vi "SRV_PM_Receive State Machine.vi"(7 "Cancelled?":bool, 8 "error in (no error)":errorcluster, 9 "SRV_Packets queue":refnum<queue>, 10 "TCP Read semaphore":T1, 11 "SRV IP Address":string) -> (0 "error out":errorcluster)   [LabVIEW 2009]
doc: "Author: Mike Schultz (LogicPD, Inc)"
uses:
  SRV_PM_Packet.ctl
  Support/SRV_Command-Data Queue Data Type.ctl
  SRV_PM_Receive State Machine Local Data.ctl
  TCP_Communication/SRV_TCP Settings.ctl
  TCP_Communication/SRV_Package Methods.ctl
  <vilib>/Utility/error.llb/DialogType.ctl
panel:
  in  "reset max 3":bool
  out "Evals max":i32
  out "Eval in a row":i32
  out "get ref ms":u32
  out "sema ms":u32
  out "Read 1 ms":u32
  in  "Delay Before Read (ms)":u32
  in  "reset max 2":bool
  out "new size max":i32
  in  "reset max":bool
  out "WIP Size max":i32
  out "Trim ms":u32
  out "New Packet Data size":i32
  out "Build ms":u32
  out "WIP Size":i32
  out "Eval ms":u32
  out "Read ms":u32
  out "Loop ms":u32
  out "ms since last ad":u32
  out "# elements in queue":i32
  out "i":i32
  out "Command History":string[](array[string])
  out "Command":string
  out "Packet Complete?":bool
  out "New Packet Data":u8[](array[numeric]) format="%.0x"
  out "Packet":T2 {"Packet Data" format="%.0x"}
  in  "Use Debug New Packet Data?":bool
  in  "New Packet Data":u8[](array[numeric]) format="%.0x"
  # "Read"
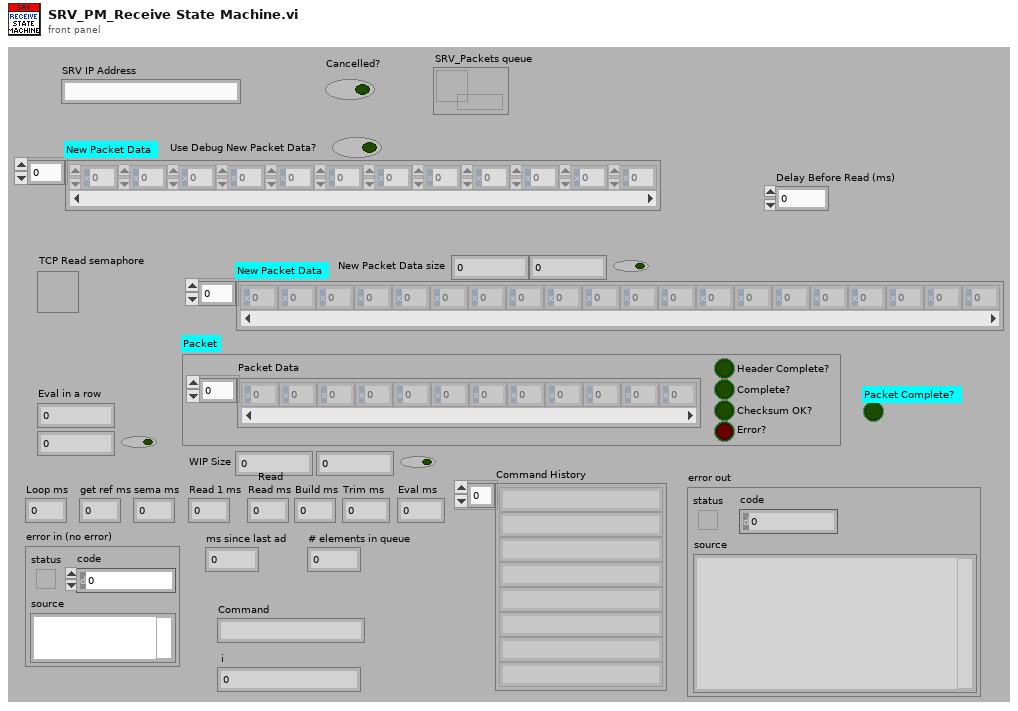
[diagram p1: front panel]
types:
  T1 = typedef "Semaphore RefNum" = refnum<k1>
  T2 = typedef "SRV_PM_Packet.ctl" = cluster{"Packet Data":u8[], "Header Complete?":bool, "Complete?":bool, "Checksum OK?":bool, "Error?":bool}
  T3 = typedef "SRV_PM_Receive State Machine Local Data.ctl" = cluster{"Packet Data WIP":u8[], "New Packet Data":u8[], "Complete Packet":T2, "SRV IP Address":string, "TCP Read semaphore":T1, "SRV_Packets queue":refnum<queue>, "Evals in a row":i32}
  T4 = typedef "SRV_Command-Data Queue Data Type.ctl" = cluster{"Command":string, "Data":variant}
  T5 = typedef "SRV_TCP Settings.ctl" = cluster{"Method":T6, "bytes to read":i32, "timeout ms (1000)":i32}
  T6 = typedef "SRV_Package Methods.ctl" = enum16{"General", "Standard", "CRLF", "Image", "HTML"}
  T7 = typedef "DialogType.ctl" = u16
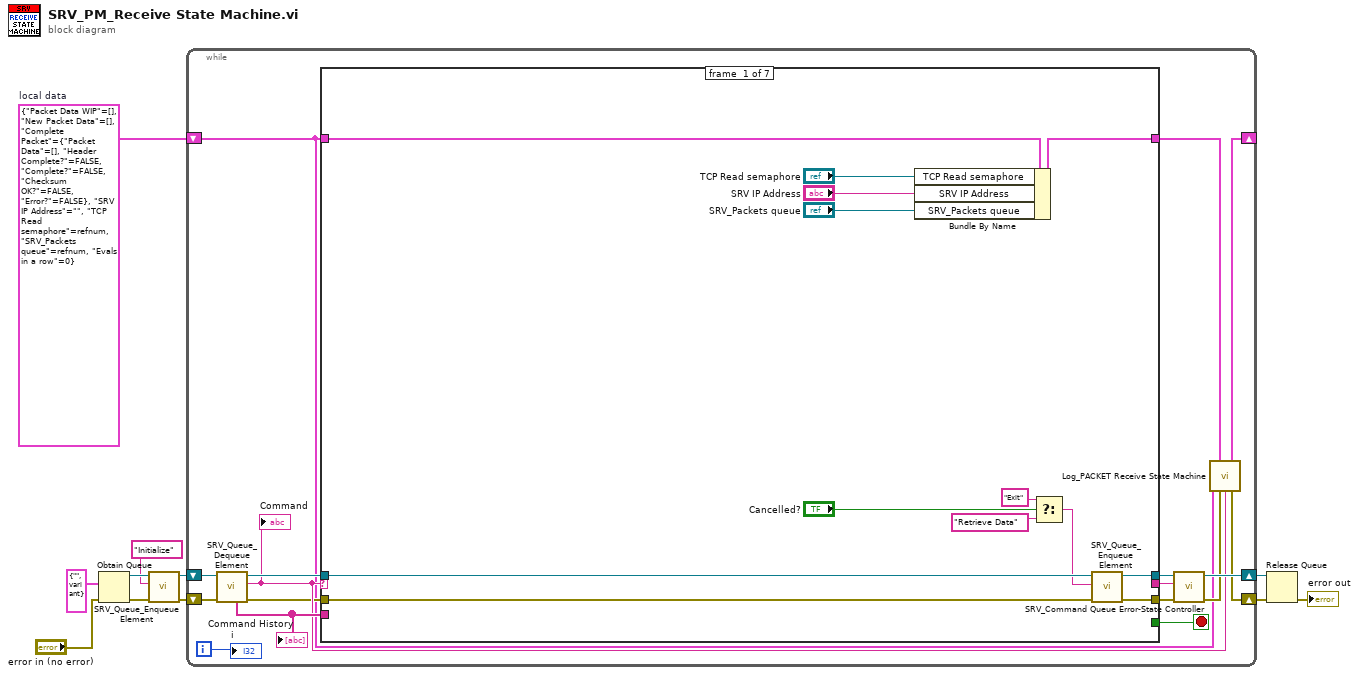
[diagram p0: block diagram]
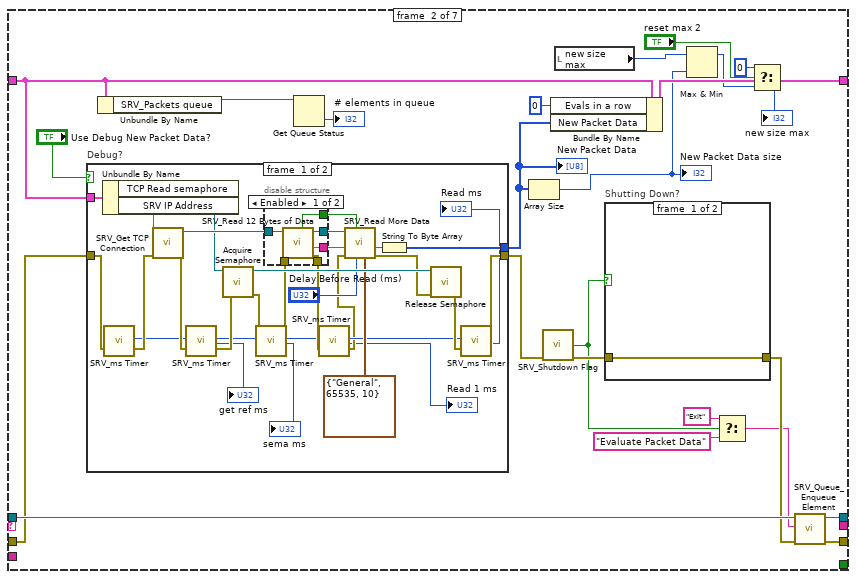
[diagram p2: hidden frame]
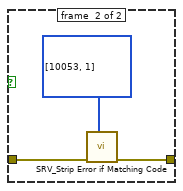
[diagram p3: hidden frame]
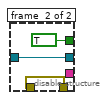
[diagram p4: hidden frame]
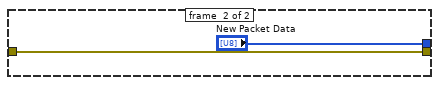
[diagram p5: hidden frame]
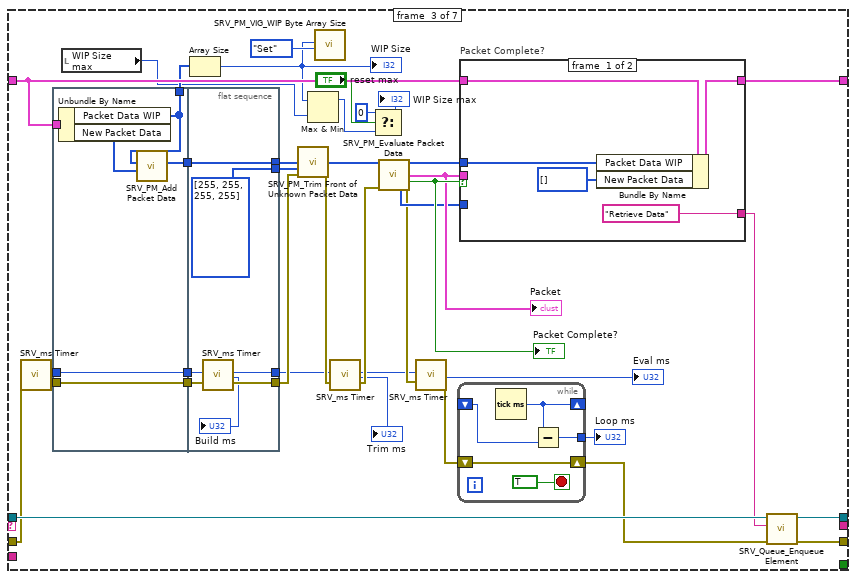
[diagram p6: hidden frame]
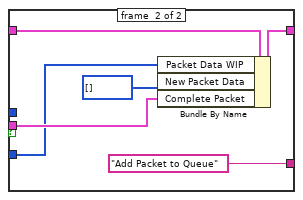
[diagram p7: hidden frame]
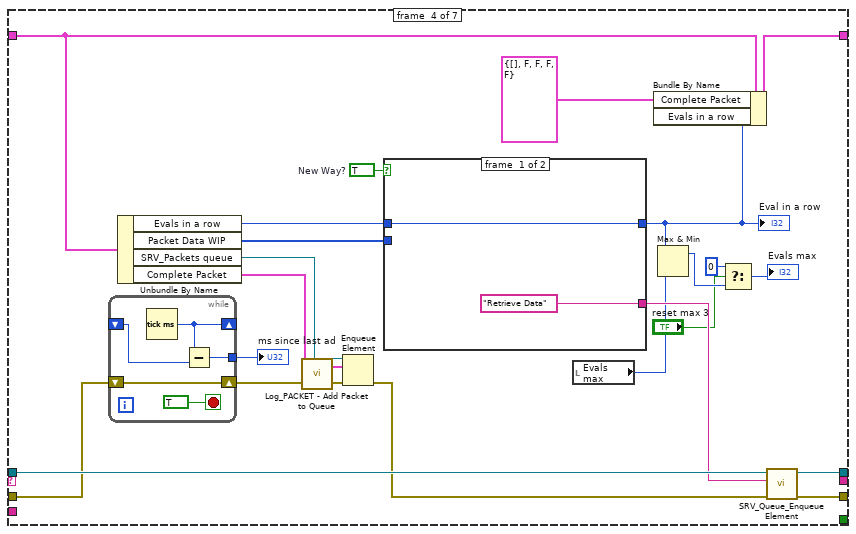
[diagram p8: hidden frame]
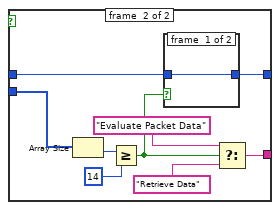
[diagram p9: hidden frame]
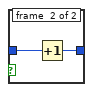
[diagram p10: hidden frame]
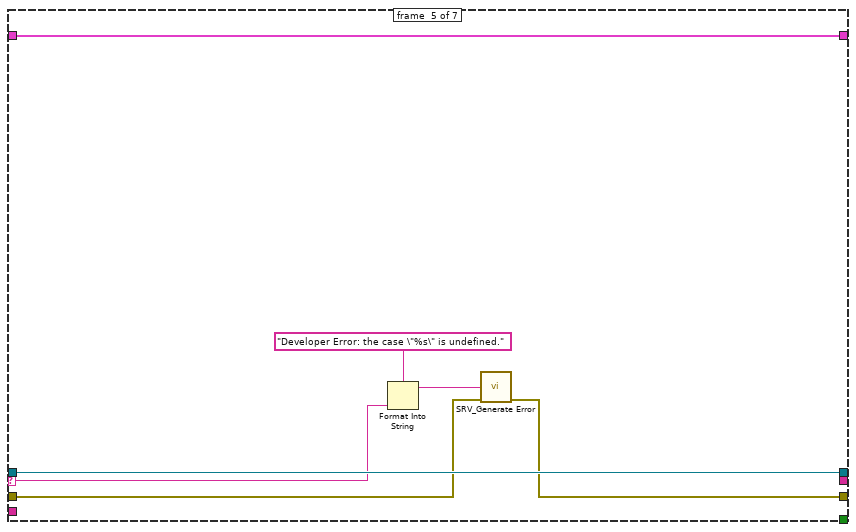
[diagram p11: hidden frame]
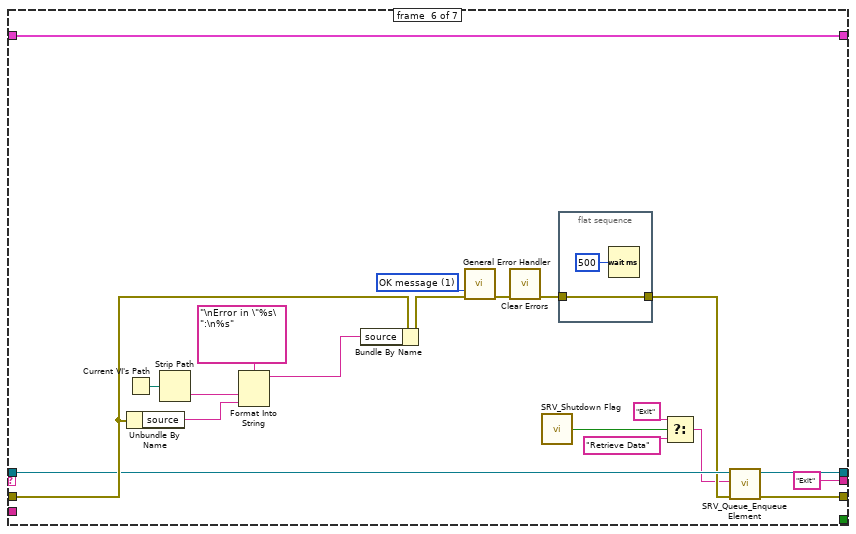
[diagram p12: hidden frame]
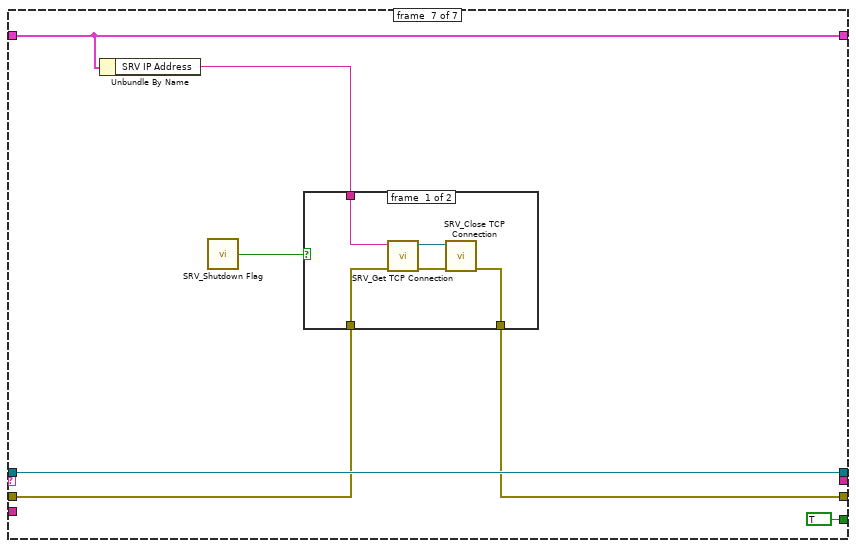
[diagram p13: hidden frame]
diagram:
  w1 = T3 {"Packet Data WIP"=[], "New Packet Data"=[], "Complete Packet"={"Packet Data"=[], "Header Complete?"=FALSE, "Complete?"=FALSE, "Checksum OK?"=FALSE, "Error?"=FALSE}, "SRV IP Address"="", "TCP Read semaphore"=refnum, "SRV_Packets queue"=refnum, "Evals in a row"=0}  # local data
  n1 = Obtain Queue(element data type=T4 {"Command"="", "Data"=variant} ("Queue Data Type"), error in (no error)="error in (no error)") -> (queue out=w10:refnum<queue>, error out=w8:errorcluster)  [unwired: 3 in, 1 out]
  n2 = call "SRV_Queue_Enqueue Element.vi"("error in (no error)"=w8, "Command"="Initialize", "Command-Data Queue"=w10) -> ("error out"=w7:errorcluster, "Command-Data Queue out"=w9:refnum<queue>)  [unwired: 6 in, 1 out]
  n3 = while {
    shift-right: [w17] -> w4
    shift-left: w7 -> [w28]
    shift-right: [w23] -> w5
    shift-left: w9 -> [w27]
    shift-right: [w14] -> _
    shift-left: w1 -> [w12]
    i -> [w19]
    stop <- w25 stop-if-true
    n4 = call "SRV_Queue_Dequeue Element.vi"("error in (no error)"=w28, "Command-Data Queue"=w27) -> ("error out"=w13:errorcluster, "Command"=w16:string, "Command-Data Queue out"=w26:refnum<queue>, "Command History"=w20:string[])  [unwired: 4 in, 2 out]
    "Command" <- w16
    "Command History" <- w20
    n5 = case shown="\"Add Packet to Queue\"" w16 {
      selector: w16 -> [_ _ _ _ w224 _ _]
      tunnel: w13 -> [w35 w61 w128 w194 w226 w238 w254]
      tunnel: [w41 w64 w148 w201 w227 w237 w255] -> w22
      tunnel: [w40 w65 w149 w202 w228 w235 w257] -> w24
      tunnel: w26 -> [w39 w63 w147 w200 w228 w236 w257]
      tunnel: [_ _ _ _ _ _ TRUE] -> w25
      tunnel: [_ _ _ _ _ "Exit" ("Error Command") _] -> w21
      tunnel: w12 -> [w38 w52 w142 w199 w222 w247 w252]
      tunnel: [w37 w62 w146 w198 w222 w247 w252] -> w15
      tunnel: w20 -> [_ _ _ _ _ _ _]
      frame #0 {
        n6 = Bundle By Name(cluster=w38, "TCP Read semaphore"="TCP Read semaphore", "SRV IP Address"="SRV IP Address", "SRV_Packets queue"="SRV_Packets queue") -> (w37:T3)
        n7 = Select(t="Exit" ("Command"), s="Cancelled?", f="Retrieve Data" ("Command")) -> (s? t:f=w31:string)
        n8 = call "SRV_Queue_Enqueue Element.vi"("error in (no error)"=w35, "Command"=w31, "Command-Data Queue"=w39) -> ("error out"=w41:errorcluster, "Command-Data Queue out"=w40:refnum<queue>)  [unwired: 6 in, 1 out]
      }
      frame #1 {
        n9 = case "Debug?" shown="False" "Use Debug New Packet Data?" {
          tunnel: w61 -> [w89 w110]
          tunnel: [w86 w110] -> w59
          tunnel: [w100 "New Packet Data"] -> w49
          tunnel: w52 -> [w94 _]
          frame #0 {
            n10 = Unbundle By Name(w94) -> ("TCP Read semaphore"=w92:T1, "SRV IP Address"=w93:string)
            n11 = call "SRV_ms Timer.vi"("error in (no error)"=w89) -> ("ms Tick"=w74:u32, "error out"=w88:errorcluster)  [unwired: 16 in, 1 out]
            n12 = call "SRV_Get TCP Connection.vi"("error in (no error)"=w88, "IP address"=w93) -> ("error out"=w78:errorcluster, "connection ID"=w95:refnum<k5>)  [unwired: 8 in]
            n13 = call "SRV_ms Timer.vi"("ms Previous Tick"=w74, "error in (no error)"=w78) -> ("ms Tick"=w73:u32, "ms Diff"=→"get ref ms":u32, "error out"=w77:errorcluster)  [unwired: 15 in]
            n14 = call <vilib>:"Acquire Semaphore.vi"("error in (no error)"=w77, "semaphore"=w92) -> ("error out"=w76:errorcluster, "semaphore out"=w91:T1)  [unwired: 3 in, 1 out]
            n15 = call "SRV_ms Timer.vi"("ms Previous Tick"=w73, "error in (no error)"=w76) -> ("ms Tick"=w72:u32, "ms Diff"=→"sema ms":u32, "error out"=w75:errorcluster)  [unwired: 15 in]
            n16 = disable-structure shown="Enabled" {
              disable-tunnel: [w106 TRUE ("Read More Data? (T)")] -> w99
              disable-tunnel: [w105 w108] -> w98
              disable-tunnel: [w104 _] -> w97
              disable-tunnel: w95 -> [w103 w108]
              disable-tunnel: [w102 w109] -> w81
              disable-tunnel: w75 -> [w101 w109]
              frame #0 {
                n17 = call "SRV_Read 12 Bytes of Data.vi"("error in (no error)"=w101, "SRV In"=w103) -> ("error out"=w102:errorcluster, "Data out"=w104:string, "SRV Out"=w105:refnum<k5>, "Read more data"=w106:bool)  [unwired: 6 in]
              }
              frame #1 {
              }
            }
            n18 = call "SRV_ms Timer.vi"("ms Previous Tick"=w72, "error in (no error)"=w81) -> ("ms Tick"=w82:u32, "ms Diff"=→"Read 1 ms":u32, "error out"=w80:errorcluster)  [unwired: 15 in]
            n19 = call "SRV_Read More Data.vi"("TCP Settings"=T5 {"Method"=enum."General", "bytes to read"=65535, "timeout ms (1000)"=10}, "Delay Before Read (10ms)"="Delay Before Read (ms)", "Read More Data? (T)"=w99, "error in (no error)"=w80, "Data in"=w97, "Connection ID"=w98) -> ("error out"=w90:errorcluster, "Data out"=w96:string)  [unwired: 3 in, 1 out]
            n20 = String To Byte Array(string=w96) -> (unsigned byte array=w100:u8[])
            n21 = call <vilib>:"Release Semaphore.vi"("error in (no error)"=w90, "semaphore"=w91) -> ("error out"=w87:errorcluster)  [unwired: 4 in, 1 out]
            n22 = call "SRV_ms Timer.vi"("ms Previous Tick"=w82, "error in (no error)"=w87) -> ("ms Diff"=→"Read ms":u32, "error out"=w86:errorcluster)  [unwired: 15 in, 1 out]
          }
          frame #1 {
          }
        }
        "New Packet Data" <- w49
        n23 = Unbundle By Name(w52) -> ("SRV_Packets queue"=w51:refnum<queue>)
        n24 = Get Queue Status(queue=w51) -> (# elements in queue=→"# elements in queue":i32)  [unwired: 2 in, 7 out]
        n25 = Array Size(array=w49) -> (size(s)=w45:i32)
        "New Packet Data size" <- w45
        n26 = call "SRV_Shutdown Flag.vi"("error in (no error)"=w59) -> ("Shutdown Flag out"=w53:bool, "error out"=w58:errorcluster)  [unwired: 13 in]
        n27 = Bundle By Name(cluster=w52, "Evals in a row"=0, "New Packet Data"=w49) -> (w62:T3)
        n28 = local read "new size max"() -> (w46:i32)
        n29 = case "Shutting Down?" shown="True" w53 {
          tunnel: w58 -> [w66 w69]
          tunnel: [w66 w68] -> w57
          frame #0 {
          }
          frame #1 {
            n30 = call "SRV_Strip Error if Matching Code.vi"("error in (no error)"=w69, "Strip Codes"=i32[] [10053, 1]) -> ("error out"=w68:errorcluster)  [unwired: 8 in]
          }
        }
        n31 = Max & Min(x=w46, y=w45) -> (max(x,y)=w48:i32)  [unwired: 1 out]
        n32 = Select(t="Exit" ("Command"), s=w53, f="Evaluate Packet Data" ("Command")) -> (s? t:f=w55:string)
        n33 = Select(t=0, s="reset max 2", f=w48) -> (s? t:f=→"new size max":i32)
        n34 = call "SRV_Queue_Enqueue Element.vi"("error in (no error)"=w57, "Command"=w55, "Command-Data Queue"=w63) -> ("error out"=w64:errorcluster, "Command-Data Queue out"=w65:refnum<queue>)  [unwired: 6 in, 1 out]
      }
      frame #2 {
        n35 = call "SRV_ms Timer.vi"("error in (no error)"=w128) -> ("ms Tick"=w126:u32, "error out"=w127:errorcluster)  [unwired: 16 in, 1 out]
        n36 = flat-sequence {
          tunnel: w142 -> [w155]
          tunnel: [w151] -> w133
          tunnel: [w150] -> w132
          tunnel: [w154] -> w130
          tunnel: [w152] -> w129
          tunnel: w127 -> [w151]
          tunnel: w126 -> [w150]
          tunnel: [w159] -> w121
          tunnel: [w158] -> w124
          tunnel: w133 -> [w161]
          tunnel: w132 -> [w160]
          tunnel: [w162] -> w131
          tunnel: w129 -> [w162]
          tunnel: [u8[] [255, 255, 255, 255] ("Search")] -> w125
          frame #0 {
            n37 = Unbundle By Name(w155) -> ("Packet Data WIP"=w154:u8[], "New Packet Data"=w153:u8[])
            n38 = call "SRV_PM_Add Packet Data.vi"("New Packet Data"=w153, "Packet Data"=w154) -> ("Packet Data out"=w152:u8[])  [unwired: 9 in]
          }
          frame #1 {
            n39 = call "SRV_ms Timer.vi"("ms Previous Tick"=w160, "error in (no error)"=w161) -> ("ms Tick"=w159:u32, "ms Diff"=→"Build ms":u32, "error out"=w158:errorcluster)  [unwired: 15 in]
          }
        }
        n40 = local read "WIP Size max"() -> (w118:i32)
        n41 = Array Size(array=w130) -> (size(s)=w112:i32)
        "WIP Size" <- w112
        n42 = call "SRV_PM_Trim Front of Unknown Packet Data.vi"("1D Array"=w131, "Search"=w125, "error in (no error)"=w124) -> ("Trimmed 1D Array"=w140:u8[], "error out"=w123:errorcluster)  [unwired: 11 in]
        n43 = Max & Min(x=w112, y=w118) -> (max(x,y)=w115:i32)  [unwired: 1 out]
        n44 = call "SRV_PM_VIG_WIP Byte Array Size.vi"("Method (Get)"=enum16{"Get", "Set"}."Set", "WIP Size"=w112) -> ()  [unwired: 8 in, 2 out]
        n45 = call "SRV_ms Timer.vi"("ms Previous Tick"=w121, "error in (no error)"=w123) -> ("ms Tick"=w120:u32, "ms Diff"=→"Trim ms":u32, "error out"=w122:errorcluster)  [unwired: 15 in]
        n46 = Select(t=0, s="reset max", f=w115) -> (s? t:f=→"WIP Size max":i32)
        n47 = call "SRV_PM_Evaluate Packet Data.vi"("Packet Data"=w140, "error in (no error)"=w122) -> ("Packet Data dup"=w145:u8[], "Packet"=w143:T2, "Packet Complete?"=w144:bool, "Extra Bytes"=w139:u8[], "error out"=w136:errorcluster)  [unwired: 9 in]
        "Packet" <- w143
        "Packet Complete?" <- w144
        n48 = call "SRV_ms Timer.vi"("ms Previous Tick"=w120, "error in (no error)"=w136) -> ("ms Diff"=→"Eval ms":u32, "error out"=w135:errorcluster)  [unwired: 15 in, 1 out]
        n49 = while {
          shift-right: [w165] -> _
          shift-left: _ -> [w164]
          shift-right: [w166] -> w138
          shift-left: w135 -> [w166]
          tunnel: [w163] -> w137
          stop <- TRUE stop-if-true
          n50 = Tick Count (ms)() -> (millisecond timer value=w165:u32)
          n51 = Subtract(x=w165, y=w164) -> (x-y=w163:u32)
        }
        "Loop ms" <- w137
        n52 = case "Packet Complete?" shown="True" w144 {
          tunnel: w142 -> [w171 w177]
          tunnel: [w172 w178] -> w146
          tunnel: w145 -> [w170 _]
          tunnel: w143 -> [_ w176]
          tunnel: ["Retrieve Data" ("Command") "Add Packet to Queue" ("Command")] -> w141
          tunnel: w139 -> [_ w173]
          frame #0 {
            n53 = Bundle By Name(cluster=w171, "Packet Data WIP"=w170, "New Packet Data"=u8[] []) -> (w172:T3)
          }
          frame #1 {
            n54 = Bundle By Name(cluster=w177, "Packet Data WIP"=w173, "New Packet Data"=u8[] [], "Complete Packet"=w176) -> (w178:T3)
          }
        }
        n55 = call "SRV_Queue_Enqueue Element.vi"("error in (no error)"=w138, "Command"=w141, "Command-Data Queue"=w147) -> ("error out"=w148:errorcluster, "Command-Data Queue out"=w149:refnum<queue>)  [unwired: 6 in, 1 out]
      }
      frame #3 {
        w191 = TRUE  # New Way?
        n56 = while {
          shift-right: [w219] -> _
          shift-left: _ -> [w218]
          shift-right: [w220] -> w180
          shift-left: w194 -> [w220]
          tunnel: [w217] -> w193
          stop <- TRUE stop-if-true
          n57 = Tick Count (ms)() -> (millisecond timer value=w219:u32)
          n58 = Subtract(x=w219, y=w218) -> (x-y=w217:u32)
        }
        "ms since last ad" <- w193
        n59 = Unbundle By Name(w199) -> ("Evals in a row"=w189:i32, "Packet Data WIP"=w192:u8[], "SRV_Packets queue"=w195:refnum<queue>, "Complete Packet"=w182:T2)
        n60 = call "Log_PACKET - Add Packet to Queue.vi"("Complete Packet"=w182, "error in (no error)"=w180) -> ("Complete Packet dup"=w181:T2, "error out"=w179:errorcluster)  [unwired: 12 in]
        n61 = Enqueue Element(queue=w195, element=w181, error in (no error)=w179) -> (error out=w196:errorcluster)  [unwired: 1 in, 2 out]
        n62 = case shown="True" w191 {
          tunnel: w192 -> [_ w213]
          tunnel: ["Retrieve Data" ("Command") w208] -> w190
          tunnel: w189 -> [w203 w206]
          tunnel: [w203 w205] -> w183
          frame #0 {
          }
          frame #1 {
            n63 = Array Size(array=w213) -> (size(s)=w212:i32)
            n64 = Greater Or Equal?(x=w212, y=14) -> (x >= y?=w207:bool)
            n65 = case shown="True" w207 {
              tunnel: w206 -> [w214 w216]
              tunnel: [w214 w215] -> w205
              frame #0 {
              }
              frame #1 {
                n66 = Increment(x=w216) -> (x+1=w215:i32)
              }
            }
            n67 = Select(t="Evaluate Packet Data" ("Command"), s=w207, f="Retrieve Data" ("Command")) -> (s? t:f=w208:string)
          }
        }
        "Eval in a row" <- w183
        n68 = local read "Evals max"() -> (w184:i32)
        n69 = Bundle By Name(cluster=w199, "Complete Packet"=T2 {"Packet Data"=[], "Header Complete?"=FALSE, "Complete?"=FALSE, "Checksum OK?"=FALSE, "Error?"=FALSE}, "Evals in a row"=w183) -> (w198:T3)
        n70 = Max & Min(x=w183, y=w184) -> (max(x,y)=w188:i32)  [unwired: 1 out]
        n71 = Select(t=0, s="reset max 3", f=w188) -> (s? t:f=→"Evals max":i32)
        n72 = call "SRV_Queue_Enqueue Element.vi"("error in (no error)"=w196, "Command"=w190, "Command-Data Queue"=w200) -> ("error out"=w201:errorcluster, "Command-Data Queue out"=w202:refnum<queue>)  [unwired: 6 in, 1 out]
      }
      frame #4 {
        n73 = Format Into String(format string="Developer Error: the case \"%s\" is undefined.", w224) -> (resulting string=w225:string)  [unwired: 2 in, 1 out]
        n74 = call "SRV_Generate Error.vi"("Message"=w225, "error in (no error)"=w226) -> ("error out"=w227:errorcluster)  [unwired: 13 in]
      }
      frame #5 {
        w246 = T7 1 items=["no dialog", "OK message", "continue or stop message", "OK message + warnings", "continue/stop + warnings"] ("type of dialog (OK msg:1)")
        n75 = Current VI's Path() -> (path=w244:path)
        n76 = Unbundle By Name(w238) -> ("source"=w242:string)
        n77 = Strip Path(path=w244) -> (name=w243:string)  [unwired: 1 out]
        n78 = Format Into String(format string="\nError in \"%s\":\n%s", w243, w242) -> (resulting string=w240:string)  [unwired: 2 in, 1 out]
        n79 = Bundle By Name(cluster=w238, "source"=w240) -> (w241:errorcluster)
        n80 = call <vilib>:"General Error Handler.vi"("type of dialog (OK msg:1)"=w246, "error in (no error)"=w241) -> ("error out"=w239:errorcluster)  [unwired: 9 in, 4 out]
        n81 = call <vilib>:"Clear Errors.vi"("error in (no error)"=w239) -> ("error out"=w234:errorcluster)  [unwired: 6 in]
        n82 = call "SRV_Shutdown Flag.vi"() -> ("Shutdown Flag out"=w232:bool)  [unwired: 14 in, 1 out]
        n83 = flat-sequence {
          tunnel: w234 -> [w250]
          tunnel: [w250] -> w233
          frame #0 {
            n84 = Wait (ms)(milliseconds to wait=u32 500) -> ()  [unwired: 1 out]
          }
        }
        n85 = Select(t="Exit" ("Command"), s=w232, f="Retrieve Data" ("Command")) -> (s? t:f=w230:string)
        n86 = call "SRV_Queue_Enqueue Element.vi"("error in (no error)"=w233, "Command"=w230, "Command-Data Queue"=w236) -> ("error out"=w237:errorcluster, "Command-Data Queue out"=w235:refnum<queue>)  [unwired: 6 in, 1 out]
      }
      frame #6 {
        n87 = Unbundle By Name(w252) -> ("SRV IP Address"=w253:string)
        n88 = call "SRV_Shutdown Flag.vi"() -> ("Shutdown Flag out"=w251:bool)  [unwired: 14 in, 1 out]
        n89 = case shown="False" w251 {
          tunnel: [w262 w263] -> w255
          tunnel: w254 -> [w259 w263]
          tunnel: w253 -> [w258 _]
          frame #0 {
            n90 = call "SRV_Get TCP Connection.vi"("error in (no error)"=w259, "IP address"=w258) -> ("error out"=w260:errorcluster, "connection ID"=w261:refnum<k5>)  [unwired: 8 in]
            n91 = call "SRV_Close TCP Connection.vi"("error in"=w260, "connection ID"=w261) -> ("error out"=w262:errorcluster)  [unwired: 9 in]
          }
          frame #1 {
          }
        }
      }
    }
    n92 = call "SRV_Command Queue Error-State Controller.vi"("error in (no error)"=w22, "Error Command"=w21, "Command-Data Queue"=w24) -> ("error out"=w18:errorcluster, "Command-Data Queue out"=w23:refnum<queue>)  [unwired: 7 in]
    n93 = call "Log_PACKET Receive State Machine.vi"("Receive State Machine Local Data"=w15, "Receive State Machine Local Data PREVIOUS"=w12, "error in (no error)"=w18, "Command"=w16) -> ("Receive State Machine Local Data dup"=w14:T3, "error out"=w17:errorcluster)  [unwired: 10 in]
    "i" <- w19
  }
  n94 = Release Queue(queue=w5, error in (no error)=w4) -> (error out=→"error out":errorcluster)  [unwired: 1 in, 2 out]
